vi "Untitled 1.vi"() -> ()   [LabVIEW 2014]
panel:
  out "transposed array":dbl[][](array[numeric])
  in  "Array 3":dbl[](array[numeric])
  in  "Array":dbl[][](array[numeric])
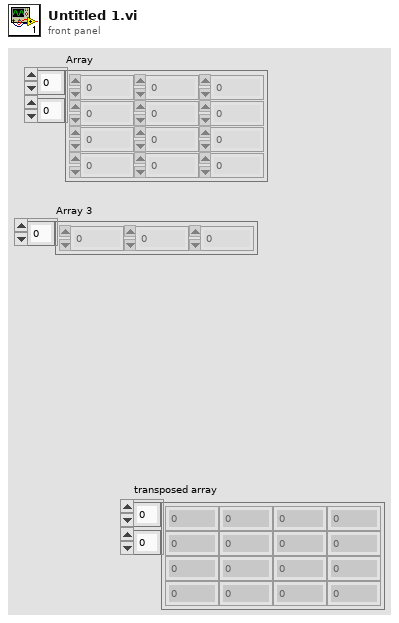
[diagram p1: front panel]
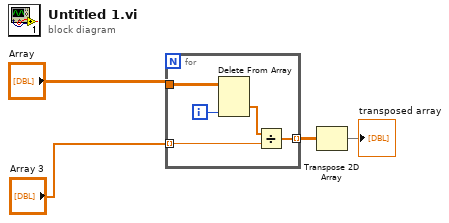
[diagram p0: block diagram]
diagram:
  n1 = for {
    tunnel: "Array" -> [w9]
    tunnel: "Array 3" -> [w7] mode=indexing
    tunnel: [w6] -> w2 mode=indexing
    i -> [w5]
    n2 = Delete From Array(array=w9, index (col)=w5) -> (deleted portion=w8:dbl[])  [unwired: 2 in, 1 out]
    n3 = Divide(x=w8, y=w7) -> (x/y=w6:dbl[])
  }
  n4 = Transpose 2D Array(2D array=w2) -> (transposed array=→"transposed array":dbl[][])
